vi "irr-sunrise-calc.vi"(8 "error in":errorcluster, 11 "Time Stamp":timestamp format="%<%x %.3X>T") -> (0 "error out":errorcluster, 1 "(T) Day (F) Night":bool, 2 "(T) Nutrients (F) Water":bool, 3 "Irrigation Time":bool)   [LabVIEW 2024]
panel:
  out "Fertilization":timestamp format="%<%x %.3X>T"
  out "Irrigation":timestamp format="%<%x %.3X>T"
  out "Sunrise":timestamp format="%<%x %.3X>T"
  out "Solar Elevation Graph":waveform(dbl)(graph)
  out "Sunset":timestamp format="%<%x %.3X>T"
  # "sunrise+60\nsunset-120"
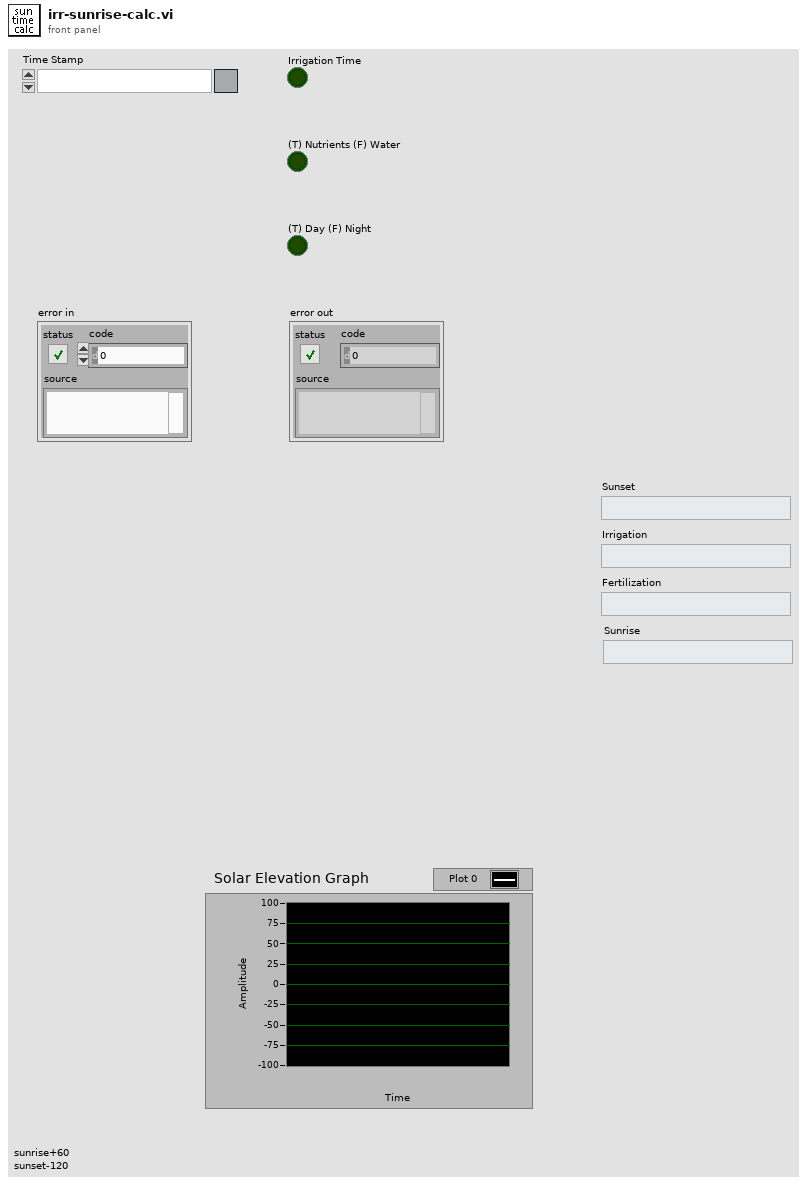
[diagram p1: front panel]
types:
  T1 = cluster{"Irrigation Timeout":timestamp, "Fertiliztion Timeout":timestamp}
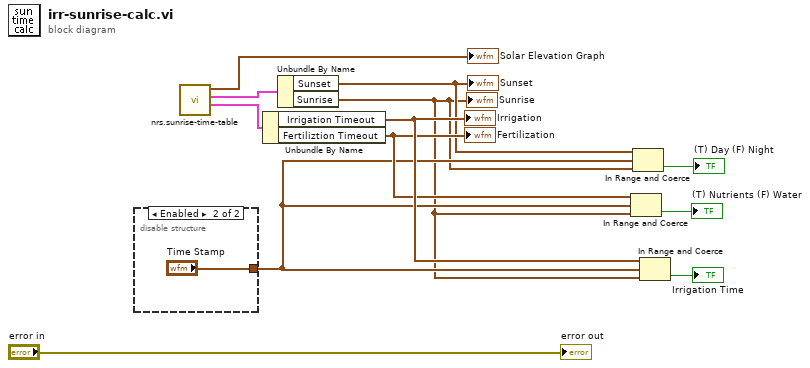
[diagram p0: block diagram]
diagram:
  n1 = disable-structure shown="Enabled" {
    disable-tunnel: [_ "Time Stamp"] -> w3
    frame Disabled {
    }
    frame Enabled {
    }
  }
  n2 = call "nrs.sunrise-time-table.vi"() -> ("Irrigation Timing"=w6:T1, "Sunrise Timing"=w5:cluster{"Sunset":timestamp, "Sunrise":timestamp}, "Solar Elevation Graph"=→"Solar Elevation Graph":waveform(dbl))  [unwired: 9 in]
  n3 = Unbundle By Name(w6) -> ("Irrigation Timeout"=w8:timestamp, "Fertiliztion Timeout"=w7:timestamp)
  "Irrigation" <- w8
  "Fertilization" <- w7
  n4 = Unbundle By Name(w5) -> ("Sunset"=w2:timestamp, "Sunrise"=w1:timestamp)
  "Sunset" <- w2
  "Sunrise" <- w1
  n5 = In Range and Coerce(upper limit=w7, x=w3, lower limit=w1) -> (In Range?=→"(T) Nutrients (F) Water":bool)  [unwired: 1 out]
  n6 = In Range and Coerce(upper limit=w2, x=w3, lower limit=w1) -> (In Range?=→"(T) Day (F) Night":bool)  [unwired: 1 out]
  n7 = In Range and Coerce(upper limit=w8, x=w3, lower limit=w1) -> (In Range?=→"Irrigation Time":bool)  [unwired: 1 out]
  "error out" <- "error in"
